vi "SetFileExtension.vi"(10 "Extension":string, 11 "File path":path) -> (3 "FilePath with Extension":path)   [LabVIEW 2017]
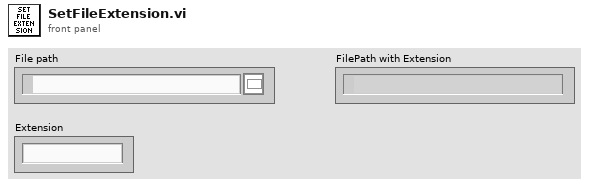
[diagram p1: front panel]
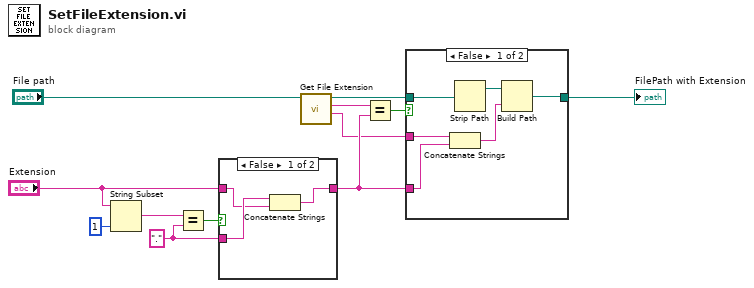
[diagram p0: block diagram]
diagram:
  w3 = "." ("y")
  n1 = String Subset(string="Extension", length (rest)=1 ("length (rest)")) -> (substring=w7:string)  [unwired: 1 in]
  n2 = Equal?(x=w7, y=w3) -> (x = y?=w5:bool)
  n3 = case shown="False" w5 {
    tunnel: "Extension" -> [w14 w16]
    tunnel: [w13 w16] -> w4
    tunnel: w3 -> [w15 _]
    frame False {
      n4 = Concatenate Strings(w15, w14) -> (w13:string)
    }
    frame True {
    }
  }
  n5 = call <vilib>:"Get File Extension.vi"("file"="File path") -> ("filename without extension"=w1:string, "lowercase file extension"=w12:string, "dup file"=w8:path)  [unwired: 6 in, 2 out]
  n6 = Equal?(x=w12, y=w4) -> (x = y?=w9:bool)
  n7 = case shown="False" w9 {
    tunnel: w8 -> [w21 w23]
    tunnel: [w18 w23] -> w10
    tunnel: w1 -> [w22 _]
    tunnel: w4 -> [w17 _]
    frame False {
      n8 = Concatenate Strings(w22, w17) -> (w19:string)
      n9 = Strip Path(path=w21) -> (stripped path=w20:path)  [unwired: 1 out]
      n10 = Build Path(base path=w20, name or relative path=w19) -> (appended path=w18:path)
    }
    frame True {
    }
  }
  "FilePath with Extension" <- w10
